vi "Test.vi"(8 "error in (no error)":errorcluster, 11 "SLSC Interface In":refnum<class "SLSC Interface.lvclass">) -> (0 "error out":errorcluster, 2 "Numeric":i32, 3 "SLSC Interface Out":refnum<class "SLSC Interface.lvclass">)   [LabVIEW 2015, in "SLSC Interface.lvclass"]
uses:
  SLSC Interface.lvclass
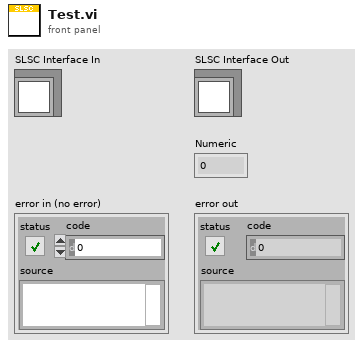
[diagram p1: front panel]
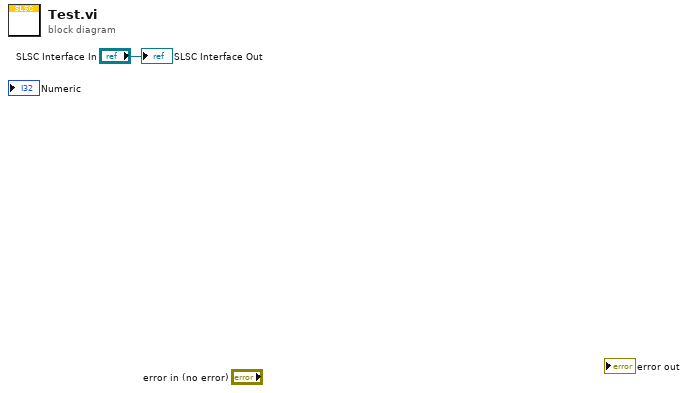
[diagram p0: block diagram]
diagram:
  "SLSC Interface Out" <- "SLSC Interface In"
